vi "Compras.vi"(8 "error in (no error)":errorcluster, 10 "Producto":string[](array[string]), 11 "UI Actor in":refnum<class "UI Actor.lvclass">) -> (0 "error out":errorcluster, 3 "UI Actor out":refnum<class "UI Actor.lvclass">)   [LabVIEW 2020, in "UI Actor.lvlib" / "UI Actor.lvclass"]
uses:
  UI Actor.lvclass
  UI Actor.lvclass/UI Actor.ctl
  UI Actor Messages/Actualizar mensaje Msg/Actualizar mensaje Msg.lvclass/Actualizar mensaje Msg.ctl
  <vilib>/ActorFramework/Message Enqueuer/Message Enqueuer.lvclass/Message Enqueuer.ctl
  UI Actor Messages/compra credito Msg/compra credito Msg.lvclass/compra credito Msg.ctl
  <vilib>/ActorFramework/Message Enqueuer/Enqueue.vi
  UI Actor Messages/Actualizar mensaje Msg/Actualizar mensaje Msg.lvclass
  C:/Program Files (x86)/National Instruments/LabVIEW 2020/vi.lib/ActorFramework/Message/Message.lvclass
  UI Actor Messages/compra credito Msg/compra credito Msg.lvclass
  <vilib>/ActorFramework/Message Priority Queue/Priority Enqueue.vi
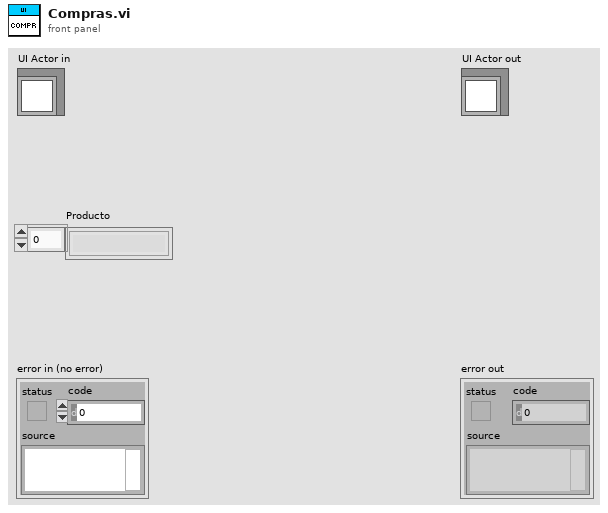
[diagram p1: front panel]
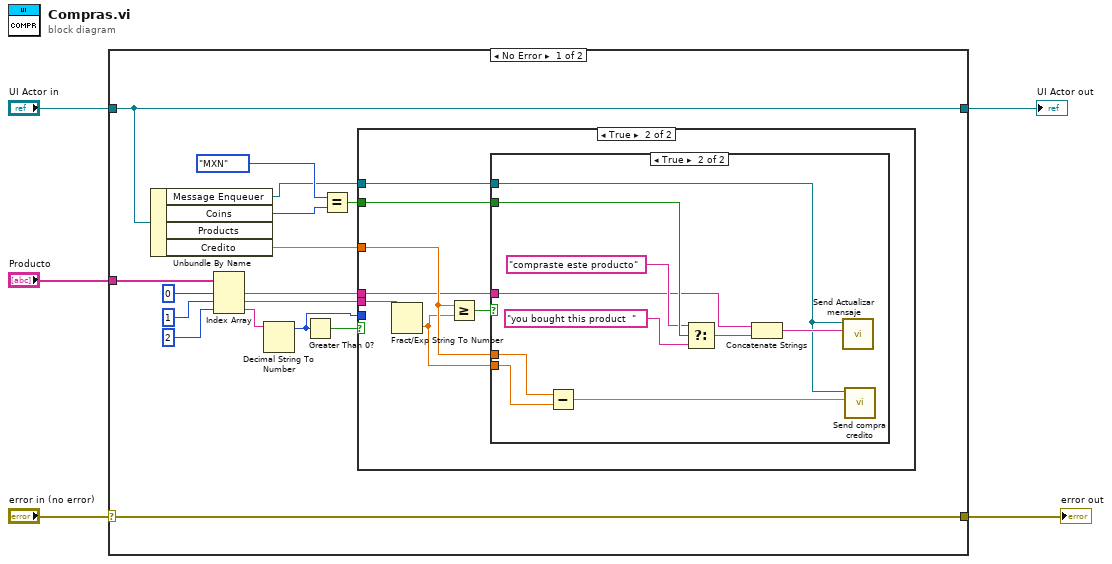
[diagram p0: block diagram]
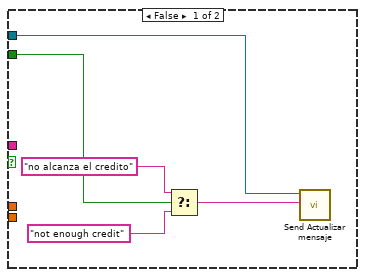
[diagram p3: hidden frame]
diagram:
  n1 = case shown="No Error" "error in (no error)" {
    selector: "error in (no error)" -> [w21 w45]
    tunnel: [w21 w45] -> w4
    tunnel: [w12 w44] -> w2
    tunnel: "UI Actor in" -> [w12 w44]
    tunnel: "Producto" -> [w15 _]
    frame No Error {
      n2 = Unbundle By Name(w12) -> ("Message Enqueuer"=w6:refnum<class "Message Enqueuer.lvclass">, "Coins"=w10:enum16{"USD", "MXN"}, "Credito"=w7:dbl)  [unwired: 1 out]
      n3 = Index Array(array=w15, index #1=0 ("index"), index #2=1 ("index"), index #3=2 ("index")) -> (element #1=w14:string, element #2=w13:string, element #3=w16:string)
      n4 = Decimal String To Number(string=w16) -> (number=w11:i32)  [unwired: 2 in, 1 out]
      n5 = Greater Than 0?(x=w11) -> (x > 0?=w17:bool)
      n6 = Equal?(x=enum16{"USD", "MXN"}."MXN", y=w10) -> (x = y?=w8:bool)
      n7 = case shown="True" w17 {
        tunnel: w14 -> [_ w24]
        tunnel: w13 -> [_ w28]
        tunnel: w7 -> [_ w26]
        tunnel: w11 -> [_ _]
        tunnel: w8 -> [_ w23]
        tunnel: w6 -> [_ w22]
        frame False {
        }
        frame True {
          n8 = Fract/Exp String To Number(string=w28) -> (number=w25:dbl)  [unwired: 3 in, 1 out]
          n9 = Greater Or Equal?(x=w26, y=w25) -> (x >= y?=w27:bool)
          n10 = case shown="True" w27 {
            tunnel: w26 -> [_ w43]
            tunnel: w25 -> [_ w42]
            tunnel: w24 -> [_ w37]
            tunnel: w23 -> [w33 w41]
            tunnel: w22 -> [w29 w34]
            frame False {
              n11 = Select(t="no alcanza el credito", s=w33, f="not enough credit") -> (s? t:f=w32:string)
              n12 = call "Send Actualizar mensaje.vi"("MSG"=w32, "Message Enqueuer"=w29) -> ()  [unwired: 8 in, 2 out]
            }
            frame True {
              n13 = Subtract(x=w43, y=w42) -> (x-y=w35:dbl)
              n14 = Select(t="compraste este producto", s=w41, f="you bought this product  ") -> (s? t:f=w38:string)
              n15 = Concatenate Strings(w37, w38) -> (w36:string)
              n16 = call "Send Actualizar mensaje.vi"("MSG"=w36, "Message Enqueuer"=w34) -> ()  [unwired: 8 in, 2 out]
              n17 = call "Send compra credito.vi"("Credito"=w35, "Message Enqueuer"=w34) -> ()  [unwired: 8 in, 2 out]
            }
          }
        }
      }
    }
    frame Error {
    }
  }
  "error out" <- w4
  "UI Actor out" <- w2
